vi "Main.vi"(11 "Module Admin":refnum<class "Delacor_lib_QMH_Module Admin.lvclass">) -> ()   [LabVIEW 2020, in "History.lvlib"]
doc: "This template is based off of the Queued Message Handler design pattern and the Queued Message Handler project template that ships with LabVIEW.\n\nThe main difference is that the queue is private to this module and communication between modules is performed via Broadcast and Request events.\n\nRequest events are wrapped in public API methods and are handled in the Event Handling Loop (EHL) of this VI. Any module can register for Broadcast events sent by this module. The EHL generates messages based on user interface actions.\n\nThe Message Handling Loop (MHL) processes messages generated by the EHL, or by other messages. The messages are string values, so new messages can be added easily to the Message Cases case structure in the MHL. Each message cluster can also provide an optional value for Message Data, which is a variant that can be converted to whatever message-specific data is required.\n_____\nBased on Delacor QMH Project Template 5.0.0.82."
uses:
  History.lvlib
  <vilib>/Delacor/Delacor QMH/Libraries/Module Admin_class/Delacor_lib_QMH_Module Admin.lvclass
  Module Data--cluster.ctl
  <vilib>/Delacor/Delacor QMH/Libraries/Message Queue_class/Delacor_lib_QMH_Message Queue.lvclass/Delacor_lib_QMH_Message Queue.ctl
  Stop Argument--cluster.ctl
  <vilib>/Delacor/Delacor QMH/Libraries/Module Admin_class/Delacor_lib_QMH_Module Admin.lvclass/Delacor_lib_QMH_Module Admin.ctl
  Agregar evento al historial Argument--cluster.ctl
  Mostrar en SubPanel Argument--cluster.ctl
  <vilib>/Delacor/Delacor QMH/Libraries/Message Queue_class/Delacor_lib_QMH_Enqueue Message (Single).vi
  <vilib>/Delacor/Delacor QMH/Libraries/Module Admin_class/Delacor_lib_QMH_Get External Launch.vi
  <vilib>/Utility/error.llb/Error Cluster From Error Code.vi
  <vilib>/ErrorRing/Error Ring.xnode
  <vilib>/Delacor/Delacor QMH/Libraries/Message Queue_class/Delacor_lib_QMH_Message Queue.lvclass
  <vilib>/Utility/miscctls.llb/LVPointTypeDef.ctl
panel:
  out "Multicolumn Listbox":i32(listbox)
  out "Lista de Eventos":string[](array[string])
  in  "CARGAR":bool
  in  "LIMPIAR":bool
  in  "Down Button":bool
  in  "Up Button":bool
  out "error out":errorcluster
  out "Status":string
  # "Histórico de Eventos"
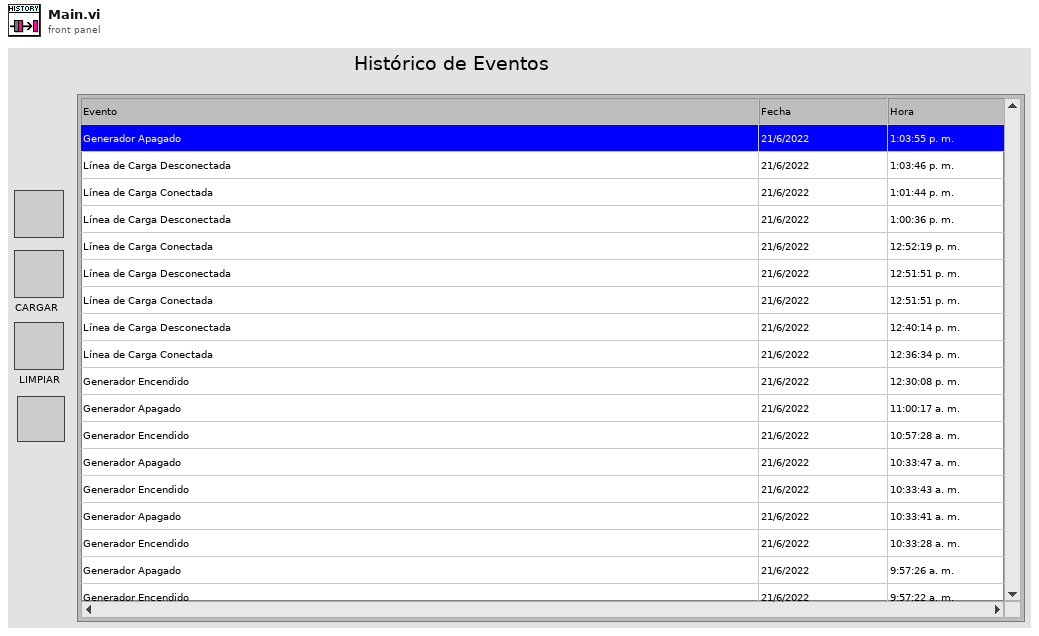
[diagram p1: front panel]
types:
  T1 = typedef "History.lvlib/Request Events--cluster.ctl" = cluster{"Stop Module":refnum<user-event>, "Show Panel":refnum<user-event>, "Hide Panel":refnum<user-event>, "Get Module Execution Status":refnum<user-event>, "Show Diagram":refnum<user-event>, "Agregar evento al historial":refnum<user-event>, "Mostrar en SubPanel":refnum<user-event>}
  T2 = typedef "History.lvlib/Module Data--cluster.ctl" = cluster{"Status":string}
  T3 = enum32{"invalid lock state", "Not Locked", "Locked (No Password)", "Password-protected"}
  T4 = typedef "History.lvlib/Stop Argument--cluster.ctl" = cluster{"Origin":string, "Exit via Stop Module Req?":bool, "Wait for Module to stop?":bool}
  T5 = typedef "History.lvlib/Agregar evento al historial Argument--cluster.ctl" = cluster{"Evento.valor":bool, "Evento.nombre":string}
  T6 = typedef "History.lvlib/Mostrar en SubPanel Argument--cluster.ctl" = cluster{"Subpanel Ref":refnum<vi>}
  T7 = enum32{"Invalid", "Standard", "Closed", "Hidden", "Minimized", "Maximized"}
  T8 = typedef "LVPointTypeDef.ctl" = cluster{"Horizontal":i16, "Vertical":i16}
  T9 = typedef "LVRowAndColumnUnsignedTypeDef.ctl" = cluster{"Row":u32, "Column":u32}
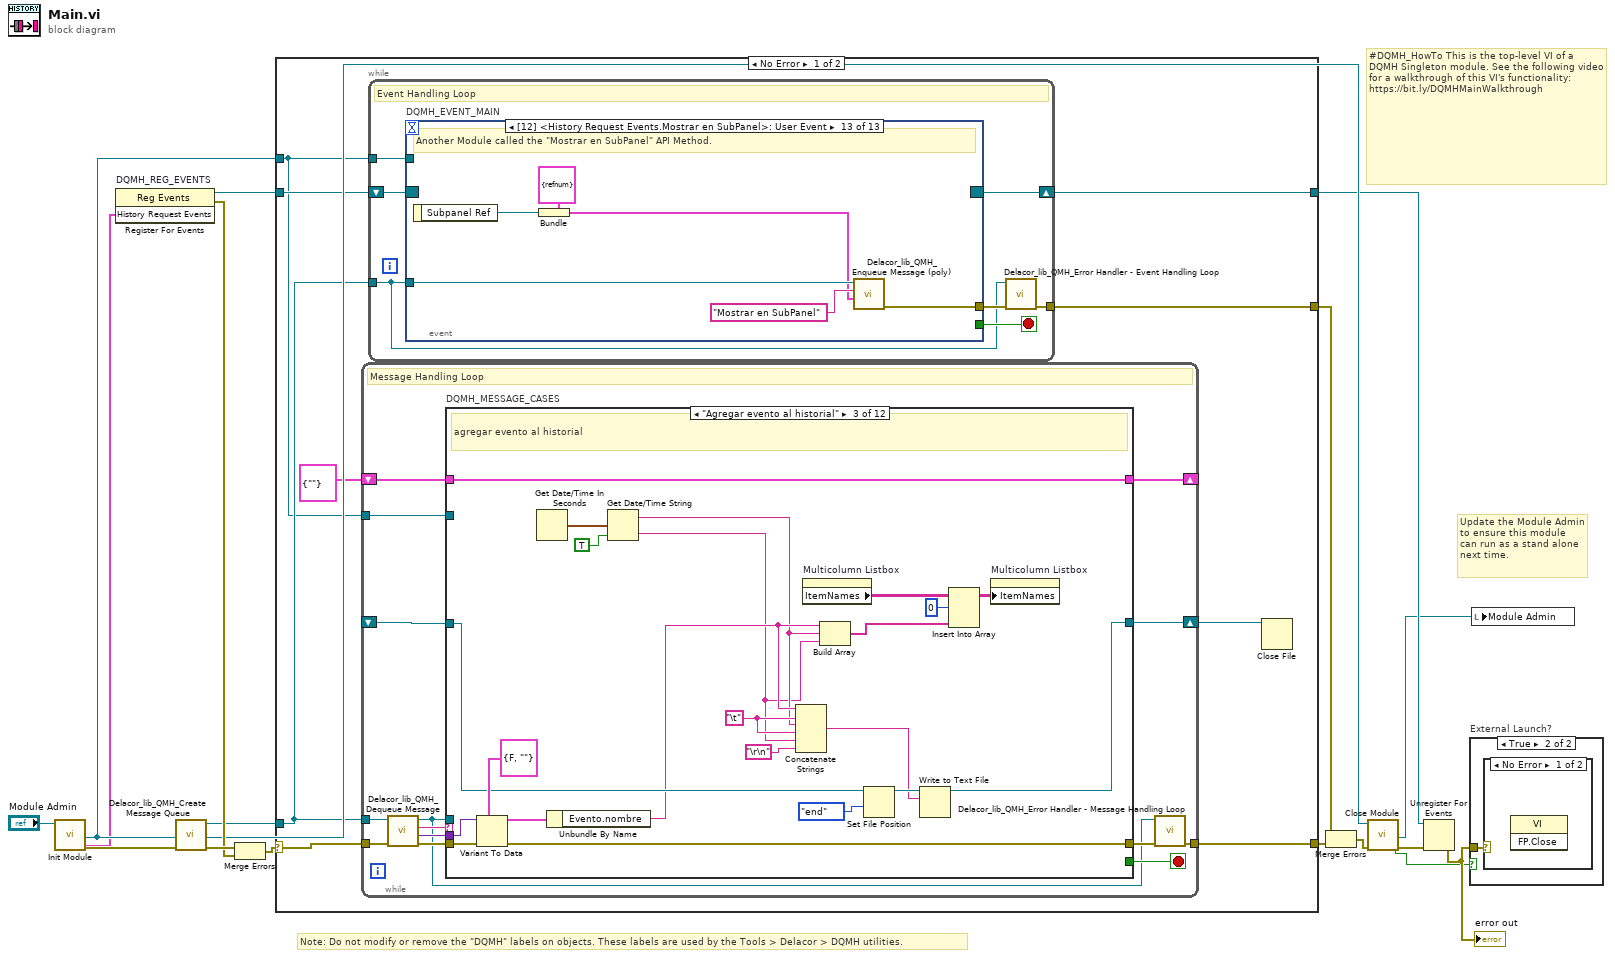
[diagram p0: block diagram]
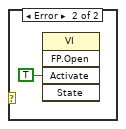
[diagram p3: hidden frame]
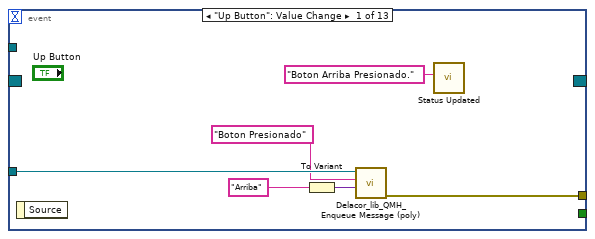
[diagram p4: hidden frame]
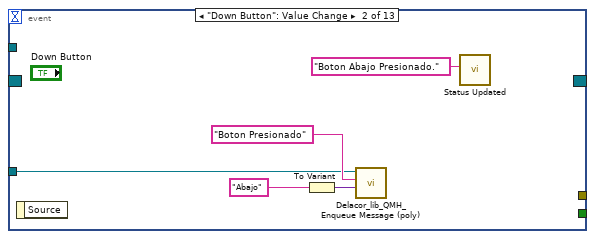
[diagram p5: hidden frame]
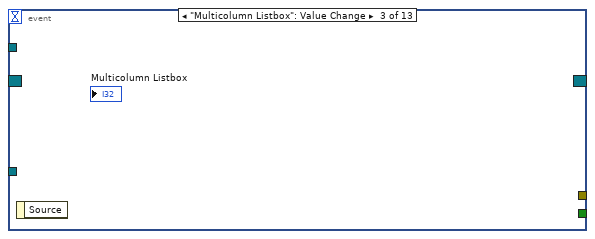
[diagram p6: hidden frame]
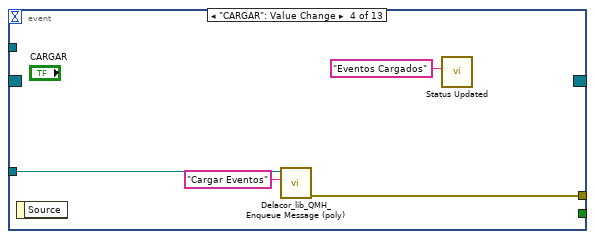
[diagram p7: hidden frame]
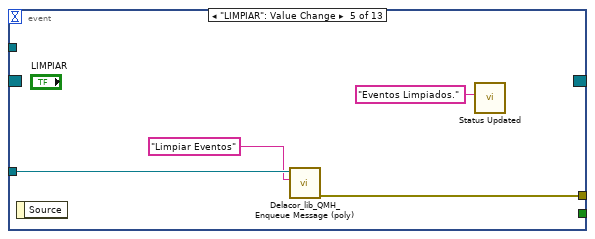
[diagram p8: hidden frame]
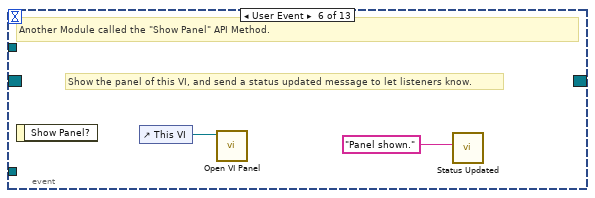
[diagram p9: hidden frame]
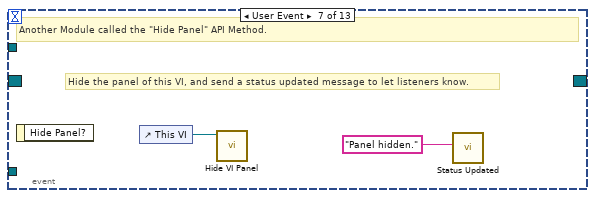
[diagram p10: hidden frame]
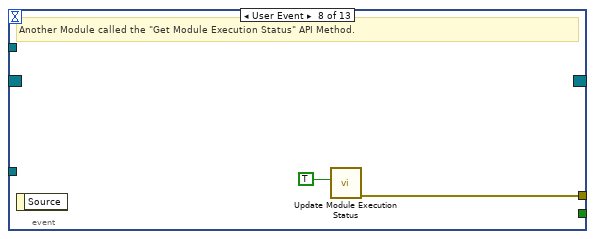
[diagram p11: hidden frame]
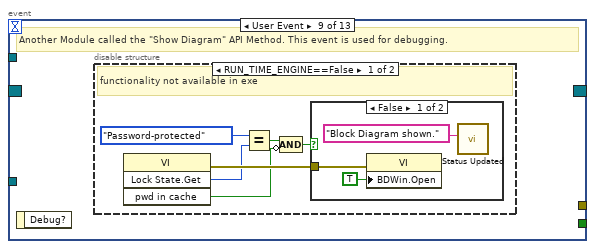
[diagram p12: hidden frame]
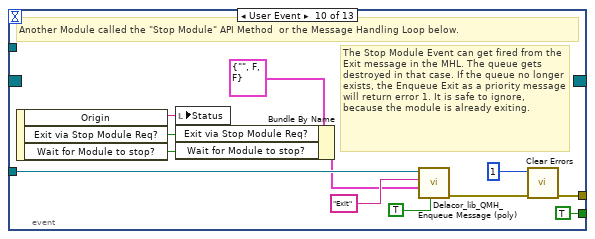
[diagram p15: hidden frame]
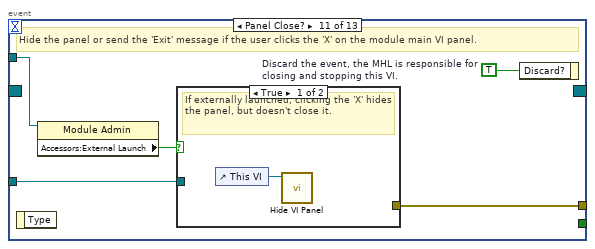
[diagram p16: hidden frame]
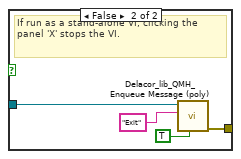
[diagram p17: hidden frame]
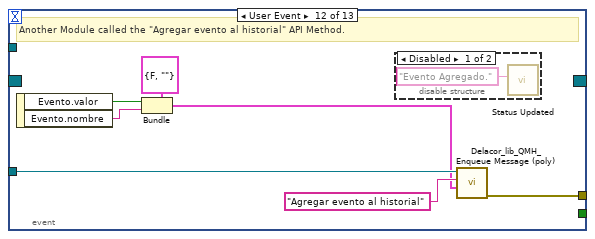
[diagram p18: hidden frame]
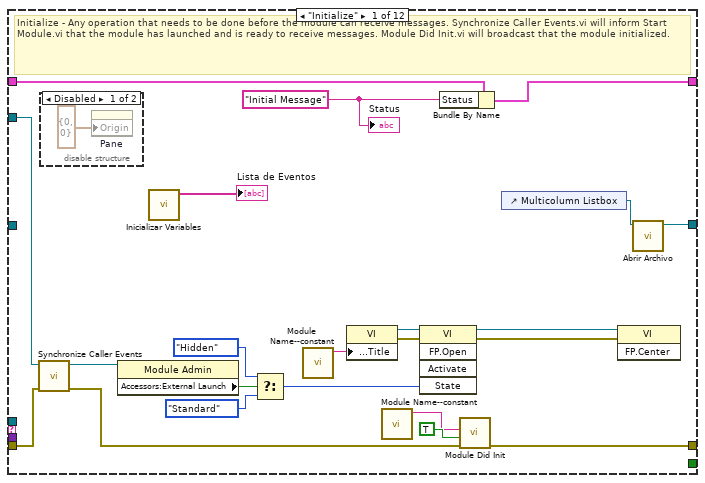
[diagram p20: hidden frame]
diagram:
  # "#DQMH_HowTo This is the top-level VI of a DQMH Singleton module. See the following video for a walkthrough of this VI's functionality: https://bit.ly/DQMHMainWalkthrough"
  # "Note: Do not modify or remove the \"DQMH\" labels on objects. These labels are used by the Tools > Delacor > DQMH utilities."
  # "Update the Module Admin to ensure this module can run as a stand alone next time."
  n1 = call "Init Module.vi"("Singleton Module Admin in"="Module Admin") -> ("error out"=w16:errorcluster, "History Request Events"=w5:T1, "Singleton Module Admin out"=w8:refnum<class "Delacor_lib_QMH_Module Admin.lvclass">)  [unwired: 8 in]
  n2 = register-events "DQMH_REG_EVENTS"(w5) -> (reference out=w6:refnum<event-registration>, error out=w9:errorcluster)  [unwired: 2 in]
  n3 = call <vilib>:"Delacor_lib_QMH_Create Message Queue.vi"("error in"=w16) -> ("error out"=w11:errorcluster, "Message Queue"=w4:refnum<class "Delacor_lib_QMH_Message Queue.lvclass">)  [unwired: 9 in]
  n4 = Merge Errors(w11, w9) -> (w10:errorcluster)
  n5 = case shown="No Error" w10 {
    selector: w10 -> [w24 w284]
    tunnel: [w26 w283] -> w17
    tunnel: [w23 w289] -> w7
    tunnel: w6 -> [w21 w289]
    tunnel: w4 -> [w20 w282]
    tunnel: [w25 _] -> w14
    tunnel: w8 -> [w19 w285]
    frame No Error {
      n6 = while {
        tunnel: w20 -> [w108]
        shift-right: [w112] -> _
        shift-left: T2 {"Status"=""} ("Data Cluster") -> [w113]
        tunnel: w24 -> [w116]
        tunnel: [w114] -> w26
        tunnel: w19 -> [w106]
        shift-right: [w105] -> w18
        shift-left: _ -> [w104]
        stop <- w111 stop-if-true
        # "Message Handling Loop"
        n7 = call-dynamic "Delacor_lib_QMH_Dequeue Message.vi"("error in"=w116, "Message Queue in"=w108) -> ("error out"=w115:errorcluster, "Message Data"=w109:variant, "Message"=w110:string, "Message Queue out"=w107:refnum<class "Delacor_lib_QMH_Message Queue.lvclass">)  [unwired: 6 in]
        n8 = case "DQMH_MESSAGE_CASES" shown="\"Agregar evento al historial\"" w110 {
          selector: w110 -> [_ _ _ _ _ _ _ _ _ _ _ w269]
          tunnel: w107 -> [_ _ _ _ _ _ _ _ _ w237 w260 _]
          tunnel: w115 -> [w137 w143 w165 w174 w178 w183 w190 w214 w232 w244 w266 w271]
          tunnel: [w135 w143 w163 w172 w177 w182 w189 w213 w232 w240 w263 w272] -> w117
          tunnel: w113 -> [w126 w142 w164 w173 w176 w181 w188 w212 w231 w239 w259 w270]
          tunnel: [w125 w142 w164 w173 w176 w181 w188 w212 w231 w239 w259 w270] -> w112
          tunnel: [_ _ _ _ _ _ _ _ _ _ w258 _] -> w111
          tunnel: w109 -> [_ _ w162 w171 _ _ _ w209 _ w238 w257 _]
          tunnel: w106 -> [w127 _ _ _ _ _ _ _ _ w236 w252 _]
          tunnel: [w118 w141 w147 _ w175 w180 w184 w211 w230 w233 w251 w267] -> w105
          tunnel: w104 -> [_ w141 w148 _ w175 w180 w186 w211 w230 w233 w251 w267]
          frame "Initialize" {
            w121 = "Initial Message" ("Initial Message")
            # "Initialize - Any operation that needs to be done before the module can receive messages. Synchronize Caller Events.vi will inform Start Module.vi that the module has launched and is ready to receive messages. Module Did Init.vi will broadcast that the module initialized."
            n9 = call "Synchronize Caller Events.vi"("error in (no error)"=w137, "Singleton Module Admin in"=w127) -> ("error out"=w136:errorcluster, "Singleton Module Admin out"=w122:refnum<class "Delacor_lib_QMH_Module Admin.lvclass">)  [unwired: 8 in]
            n10 = disable-structure shown="Disabled" {
              frame Disabled {
                n11 = property on="Pane" class="Pane"("Origin"=T8 {"Horizontal"=0, "Vertical"=0}) -> ()  [unwired: 2 in, 2 out]
              }
              frame Enabled {
              }
            }
            n12 = property class="Module Admin"(reference=w122) -> ("Accessors:External Launch"=w131:bool)  [unwired: 1 in, 2 out]
            n13 = call "Inicializar Variables.vi"() -> ("Lista de Eventos"=→"Lista de Eventos":string[])  [unwired: 11 in]
            n14 = Select(t=T7."Hidden" ("State"), s=w131, f=T7."Standard" ("State")) -> (s? t:f=w128:T7)
            n15 = call "Module Name--constant.vi"() -> ("Module Name"=w134:string)  [unwired: 11 in]
            n16 = property class="VI"("Front Panel.Title"=w134) -> (reference out=w133:refnum<vi>, error out=w139:errorcluster)  [unwired: 2 in]
            n17 = call "Module Name--constant.vi"() -> ("Module Name"=w123:string)  [unwired: 11 in]
            n18 = invoke class="VI" method="FP.Open"(reference=w133, error in=w139, "State"=w128) -> (reference out=w132:refnum<vi>, error out=w138:errorcluster)  [unwired: 2 in, 3 out]
            n19 = Bundle By Name(cluster=w126, "Status"=w121) -> (w125:T2)
            n20 = call "Module Did Init.vi"("error in (no error)"=w136, "Initialized?"=TRUE, "Origin"=w123) -> ("error out"=w135:errorcluster)  [unwired: 8 in]
            n21 = control-ref of="Multicolumn Listbox"() -> (w119:refnum<vi>)
            n22 = invoke class="VI" method="FP.Center"(reference=w132, error in=w138) -> ()  [unwired: 1 in, 3 out]
            n23 = call "Abrir Archivo.vi"("MulticolumnListbox in"=w119) -> ("Byte Stream File out"=w118:refnum<file>)  [unwired: 10 in]
            "Status" <- w121
          }
          frame "--- Module Specific ---" {
            # "Separator -- The following cases handle messages specific to this Module."
          }
          frame "Agregar evento al historial" {
            w151 = "\t"
            # "agregar evento al historial"
            n24 = Variant To Data(error in=w165, type=T5 {"Evento.valor"=FALSE, "Evento.nombre"=""} ("Agregar evento al historial Argument"), Variant=w162) -> (data=w160:T5, error out=w163:errorcluster)
            n25 = Get Date/Time In Seconds() -> (seconds since 1Jan1904=w159:timestamp)
            n26 = Unbundle By Name(w160) -> ("Evento.nombre"=w146:string)
            n27 = Get Date/Time String(seconds (now)=w159, want seconds? (F)=TRUE) -> (date string=w145:string, time string=w144:string)  [unwired: 1 in]
            n28 = Concatenate Strings(w146, w151, w145, w151, w144, "\r\n") -> (w153:string)
            n29 = property on="Multicolumn Listbox" class="MCListbox (strict)"() -> ("ItemNames"=w156:string[][])  [unwired: 2 in, 2 out]
            n30 = Build Array(w146, w145, w144) -> (w149:string[])
            n31 = Set File Position(refnum=w148, from (0:start)=enum16{"start", "end", "current"}."end") -> (refnum out=w154:refnum<file>)  [unwired: 2 in, 1 out]
            n32 = Write to Text File(file (use dialog)=w154, text=w153) -> (refnum out=w147:refnum<file>)  [unwired: 2 in, 2 out]
            n33 = Insert Into Array(array=w156, index (row)=0, new element=w149) -> (w155:string[][])  [unwired: 1 in]
            n34 = property on="Multicolumn Listbox" class="MCListbox (strict)"("ItemNames"=w155) -> ()  [unwired: 2 in, 2 out]
          }
          frame "Mostrar en SubPanel" {
            # "#CodeNeeded\n1. Configure this Message Case for handling the \"Mostrar en SubPanel\" message.\n2. Delete or edit this label when done."
            # "Mostrar el Módulo de Historial en el SubPanel del Main Module"
            n35 = Variant To Data(error in=w174, type=T6 {"Subpanel Ref"=refnum} ("Mostrar en SubPanel Argument"), Variant=w171) -> (data=w169:T6, error out=w172:errorcluster)
            n36 = Unbundle By Name(w169) -> ("Subpanel Ref"=w166:refnum<vi>)
            n37 = call "Module Name--constant.vi"() -> ("Module Name"=w167:string)  [unwired: 11 in]
            n38 = property class="VI"("Front Panel.Title"=w167) -> (reference out=w168:refnum<vi>)  [unwired: 2 in, 1 out]
            n39 = call "Insert SubPanel.vi"("VI Ref"=w168, "Subpanel Ref"=w166) -> ()  [unwired: 9 in, 1 out]
          }
          frame "---Copy This Frame---" {
            # "Duplicate this frame when creating new messages.  Change this comment in the duplicated frame to describe this message."
            n40 = Merge Errors(w178) -> (w177:errorcluster)
          }
          frame "Limpiar Eventos" {
            # "Duplicate this frame when creating new messages.  Change this comment in the duplicated frame to describe this message."
            n41 = property on="Multicolumn Listbox" class="MCListbox (strict)"("ItemNames"=string[][] [] ("Item Names")) -> ()  [unwired: 2 in, 2 out]
            n42 = Merge Errors(w183) -> (w182:errorcluster)
          }
          frame "Cargar Eventos" {
            # "Duplicate this frame when creating new messages.  Change this comment in the duplicated frame to describe this message."
            n43 = flat-sequence {
              tunnel: w186 -> [w193]
              tunnel: [w197] -> w187
              tunnel: [w191] -> w185
              tunnel: w187 -> [w203]
              tunnel: [w202] -> w184
              tunnel: w185 -> [w202]
              frame #0 {
                n44 = Set File Position(refnum=w193, from (0:start)=enum16{"start", "end", "current"}."start") -> (refnum out=w192:refnum<file>)  [unwired: 2 in, 1 out]
                n45 = Read from Text File(file (use dialog)=w192) -> (refnum out=w196:refnum<file>, text=w199:string)  [unwired: 2 in, 3 out]
                n46 = property on="Multicolumn Listbox" class="MCListbox (strict)"("ItemNames"=string[][] [] ("Array")) -> ()  [unwired: 2 in, 2 out]
                n47 = Spreadsheet String To Array(format string="%s", spreadsheet string=w199, array type (2D Dbl)=string[][] [] ("Array")) -> (array=w197:string[][])  [unwired: 1 in]
                n48 = Set File Position(refnum=w196, from (0:start)=enum16{"start", "end", "current"}."start") -> (refnum out=w191:refnum<file>)  [unwired: 2 in, 1 out]
              }
              frame #1 {
                n49 = for {
                  tunnel: w203 -> [w205] mode=indexing
                  n50 = property on="Multicolumn Listbox" class="MCListbox (strict)"() -> ("ItemNames"=w207:string[][])  [unwired: 2 in, 2 out]
                  n51 = Insert Into Array(array=w207, index (row)=0, new element=w205) -> (w206:string[][])  [unwired: 1 in]
                  n52 = property on="Multicolumn Listbox" class="MCListbox (strict)"("ItemNames"=w206) -> ()  [unwired: 2 in, 2 out]
                }
              }
            }
            n53 = Merge Errors(w190) -> (w189:errorcluster)
          }
          frame "Boton Presionado" {
            # "Duplicate this frame when creating new messages.  Change this comment in the duplicated frame to describe this message."
            n54 = Variant To Data(type="" ("Message"), Variant=w209) -> (data=w208:string)  [unwired: 1 in, 1 out]
            n55 = case shown="\"Abajo\", Default" w208 {
              frame "Abajo", Default {
                n56 = local read "Multicolumn Listbox"() -> (w218:i32)
                n57 = Greater?(x=w218, y=5) -> (0:w219:bool)
                n58 = case shown="True" w219 {
                  frame False {
                  }
                  frame True {
                    n59 = property on="Multicolumn Listbox" class="MCListbox (strict)"() -> ("TopLeft"=w222:T9)  [unwired: 2 in, 2 out]
                    n60 = Unbundle By Name(w222) -> ("Row"=w220:u32, "Column"=w224:u32)
                    n61 = Increment(x=w220) -> (x+1=w221:u32)
                    n62 = Bundle By Name(cluster=w222, "Row"=w221, "Column"=w224) -> (w223:T9)
                    n63 = property on="Multicolumn Listbox" class="MCListbox (strict)"("TopLeft"=w223) -> ()  [unwired: 2 in, 2 out]
                  }
                }
                n64 = Add(x=w218, y=1) -> (x+y=w217:i32)
                n65 = local write "Multicolumn Listbox"(w217) -> ()
              }
              frame "Arriba" {
                n66 = local read "Multicolumn Listbox"() -> (w226:i32)
                n67 = Equal To 0?(x=w226) -> (x = 0?=w229:bool)
                n68 = Subtract(x=w226, y=1) -> (x-y=w227:i32)
                n69 = Select(t=w226, s=w229, f=w227) -> (s? t:f=w228:i32)
                n70 = local write "Multicolumn Listbox"(w228) -> ()
              }
            }
            n71 = Merge Errors(w214) -> (w213:errorcluster)
          }
          frame "--- Exit and Error Handling---" {
            # "Separator - The following cases handle errors and exit messages."
          }
          frame "Error" {
            # "#CodeRecommended - If you ever change the name of this \"Error\" message, you'll need to update the name in the Check Loop Error.vi as well."
            # "#CodeRecommended - If the module is running in standalone mode (External Launch = FALSE), this code will pop up an error dialog and call the 'Exit' message if an error occurs. Add more fine-grained error handling here."
            # "Error - Check the error message data and respond accordingly. This message is sent by the \"Error Handler\" VIs at the end of each loop in this application."
            n72 = Variant To Data(error in=w244, type=errorcluster {"status"=FALSE, "code"=0, "source"=""} ("error constant"), Variant=w238) -> (data=w245:errorcluster, error out=w242:errorcluster)
            n73 = property class="Module Admin"(reference=w236) -> ("Accessors:External Launch"=w235:bool)  [unwired: 1 in, 2 out]
            n74 = call "Module Name--constant.vi"() -> ("Module Name"=w234:string)  [unwired: 11 in]
            n75 = call "Error Reported.vi"("Additional Information"=w234, "Error"=w245) -> ()  [unwired: 9 in, 1 out]
            n76 = case shown="False" w235 {
              tunnel: [w250 _] -> w241
              tunnel: w237 -> [w248 _]
              tunnel: w245 -> [w249 _]
              frame False {
                # "If the module is running standalone, then pop up an error dialog and call the \"Exit\" message."
                n77 = call <vilib>:"Simple Error Handler.vi"("error in (no error)"=w249) -> ()  [unwired: 4 in, 5 out]
                n78 = call-poly <vilib>:"Delacor_lib_QMH_Enqueue Message (poly).vi"("Priority Message? (F)"=TRUE, "Message"="Exit", "Message Queue in"=w248) -> ("error out"=w250:errorcluster)  [unwired: 7 in, 1 out]
              }
              frame True {
                # "If the module was launched externally, calling the Error Reported broadcast VI is the only action performed by the \"Error\" message. The module's caller can then process the error appropriately."
              }
            }
            n79 = Merge Errors(w242, w241) -> (w240:errorcluster)
            n80 = local write "error out"(w240) -> ()
          }
          frame "Exit" {
            w256 = 91  # 91: not all Exit messages will have an argument
            w258 = TRUE  # Stop the VI
            # "Release the message queue reference"
            # "#CodeNeeded - Add any required cleanup code here"
            # "Exit - Exit the application."
            n81 = Variant To Data(error in=w266, type=T4 {"Origin"="", "Exit via Stop Module Req?"=FALSE, "Wait for Module to stop?"=FALSE} ("Stop Argument"), Variant=w257) -> (data=w254:T4, error out=w262:errorcluster)
            n82 = call <vilib>:"Clear Errors.vi"("error in (no error)"=w262, "specific error code to clear (0: all)"=w256) -> ("error out"=w265:errorcluster)  [unwired: 4 in, 1 out]
            n83 = control-ref of="This VI"() -> (w253:refnum<vi>)
            n84 = call-dynamic "Delacor_lib_QMH_Release Message Queue.vi"("error in"=w265, "Message Queue"=w260) -> ("error out"=w264:errorcluster)  [unwired: 9 in]
            n85 = call "Handle Exit.vi"("Stop Argument"=w254, "Admin in"=w252, "VI reference"=w253) -> ("error out"=w261:errorcluster)  [unwired: 7 in, 1 out]
            n86 = Merge Errors(w264, w261) -> (w263:errorcluster)
          }
          frame Default {
            # "'Default' case only runs if there is a message that isn't defined in any of the other cases.  Output a programming error."
            n87 = call "Module Name--constant.vi"() -> ("Module Name"=w268:string)  [unwired: 11 in]
            n88 = xnode "Error Ring"("parameter 0"=w269, "parameter 1"=w268) -> ("error out"=w273:errorcluster)
            n89 = Merge Errors(w271, w273) -> (w272:errorcluster)
          }
        }
        n90 = call-dynamic "Delacor_lib_QMH_Error Handler - Message Handling Loop.vi"("error in"=w117, "Message Queue in"=w107) -> ("dup error in"=w114:errorcluster)  [unwired: 8 in, 1 out]
      }
      n91 = while {
        tunnel: w20 -> [w27]
        shift-right: [w30] -> w23
        shift-left: w21 -> [w31]
        tunnel: [w32] -> w25
        tunnel: w19 -> [w28]
        stop <- w29 stop-if-true
        # "Event Handling Loop"
        n92 = event "DQMH_EVENT_MAIN" shown="[12] <History Request Events.Mostrar en SubPanel>: User Event" {
          selector: w31 -> [_ _ _ _ _ _ _ _ _ _ _ _ _]
          dyn-events: [_ _ _ _ _ _ _ _ _ _ _ _ _] -> w30
          timeout: _ -> [_ _ _ _ _ _ _ _ _ _ _ _ _]
          tunnel: [_ _ _ _ _ _ _ _ _ TRUE ("Discard?") _ _ _] -> w29
          tunnel: w27 -> [w39 w41 _ w48 w51 _ _ _ _ w75 w82 w96 w103]
          tunnel: [w34 _ _ w45 w49 _ _ w58 _ w78 w84 w90 w98] -> w33
          tunnel: w28 -> [_ _ _ _ _ _ _ _ _ _ w81 _ _]
          event "Up Button": Value Change {
            n93 = event-data() -> ()  [unwired: 1 in, 1 out]
            n94 = To Variant(anything="Arriba" ("Message")) -> (Variant=w36:variant)
            n95 = call-poly <vilib>:"Delacor_lib_QMH_Enqueue Message (poly).vi"("Message Data"=w36, "Message"="Boton Presionado", "Message Queue in"=w39) -> ("error out"=w34:errorcluster)  [unwired: 7 in, 1 out]
            n96 = call "Status Updated.vi"("Status"="Boton Arriba Presionado.") -> ()  [unwired: 10 in, 1 out]
          }
          event "Down Button": Value Change {
            n97 = event-data() -> ()  [unwired: 1 in, 1 out]
            n98 = To Variant(anything="Abajo" ("Message")) -> (Variant=w44:variant)
            n99 = call-poly <vilib>:"Delacor_lib_QMH_Enqueue Message (poly).vi"("Message Data"=w44, "Message"="Boton Presionado", "Message Queue in"=w41) -> ()  [unwired: 7 in, 2 out]
            n100 = call "Status Updated.vi"("Status"="Boton Abajo Presionado.") -> ()  [unwired: 10 in, 1 out]
          }
          event "Multicolumn Listbox": Value Change {
            n101 = event-data() -> ()  [unwired: 1 in, 1 out]
          }
          event "CARGAR": Value Change {
            n102 = event-data() -> ()  [unwired: 1 in, 1 out]
            n103 = call-poly <vilib>:"Delacor_lib_QMH_Enqueue Message (poly).vi"("Message"="Cargar Eventos", "Message Queue in"=w48) -> ("error out"=w45:errorcluster)  [unwired: 8 in, 1 out]
            n104 = call "Status Updated.vi"("Status"="Eventos Cargados") -> ()  [unwired: 10 in, 1 out]
          }
          event "LIMPIAR": Value Change {
            n105 = event-data() -> ()  [unwired: 1 in, 1 out]
            n106 = call-poly <vilib>:"Delacor_lib_QMH_Enqueue Message (poly).vi"("Message"="Limpiar Eventos" ("Status"), "Message Queue in"=w51) -> ("error out"=w49:errorcluster)  [unwired: 8 in, 1 out]
            n107 = call "Status Updated.vi"("Status"="Eventos Limpiados.") -> ()  [unwired: 10 in, 1 out]
          }
          event User Event {
            # "Show the panel of this VI, and send a status updated message to let listeners know."
            # "Another Module called the \"Show Panel\" API Method."
            n108 = event-data() -> ()  [unwired: 1 in, 1 out]
            n109 = control-ref of="This VI"() -> (w54:refnum<vi>)
            n110 = call "Open VI Panel.vi"("VI"=w54) -> ()  [unwired: 10 in, 1 out]
            n111 = call "Status Updated.vi"("Status"="Panel shown." ("format string")) -> ()  [unwired: 10 in, 1 out]
          }
          event User Event {
            # "Hide the panel of this VI, and send a status updated message to let listeners know."
            # "Another Module called the \"Hide Panel\" API Method."
            n112 = event-data() -> ()  [unwired: 1 in, 1 out]
            n113 = control-ref of="This VI"() -> (w56:refnum<vi>)
            n114 = call "Hide VI Panel.vi"("VI"=w56) -> ()  [unwired: 10 in, 1 out]
            n115 = call "Status Updated.vi"("Status"="Panel hidden." ("format string")) -> ()  [unwired: 10 in, 1 out]
          }
          event User Event {
            # "Another Module called the \"Get Module Execution Status\" API Method."
            n116 = event-data() -> ()  [unwired: 1 in, 1 out]
            n117 = call "Update Module Execution Status.vi"("Running?"=TRUE) -> ("error out"=w58:errorcluster)  [unwired: 10 in]
          }
          event User Event {
            # "Another Module called the \"Show Diagram\" API Method. This event is used for debugging."
            n118 = event-data() -> ()  [unwired: 1 in, 1 out]
            n119 = disable-structure shown="RUN_TIME_ENGINE==False" {
              frame condition #0 (active) {
                # "functionality not available in exe"
                n120 = invoke class="VI" method="Lock State.Get"() -> (error out=w64:errorcluster, "Get Lock State"=w63:T3, "pwd in cache"=w60:bool)  [unwired: 4 in, 1 out]
                n121 = Equal?(x=T3."Password-protected", y=w63) -> (x = y?=w61:bool)
                n122 = Compound Arithmetic op=AND(w61, invert w60) -> (w59:bool)
                n123 = case shown="False" w59 {
                  tunnel: w64 -> [w67 _]
                  frame False {
                    n124 = property class="VI"(error in=w67, "BDWin.Open"=TRUE ("Block Diagram Window:Open")) -> ()  [unwired: 1 in, 2 out]
                    n125 = call "Status Updated.vi"("Status"="Block Diagram shown." ("format string")) -> ()  [unwired: 10 in, 1 out]
                  }
                  frame True {
                    # "Password-protected VI, and the password is not in the cache. Do not show the diagram."
                  }
                }
              }
              frame condition #1 {
              }
            }
          }
          event User Event {
            # "The Stop Module Event can get fired from the Exit message in the MHL. The queue gets destroyed in that case. If the queue no longer exists, the Enqueue Exit as a priority message will return error 1. It is safe to ignore, because the module is already exiting."
            # "Another Module called the \"Stop Module\" API Method  or the Message Handling Loop below."
            n126 = event-data() -> ("Origin"=w74:string, "Exit via Stop Module Req?"=w70:bool, "Wait for Module to stop?"=w69:bool)  [unwired: 1 in]
            n127 = local write "Status"(w74) -> ()
            n128 = Bundle By Name(cluster=T4 {"Origin"="", "Exit via Stop Module Req?"=FALSE, "Wait for Module to stop?"=FALSE} ("Stop Argument"), "Exit via Stop Module Req?"=w70, "Wait for Module to stop?"=w69) -> (w68:T4)
            n129 = call-poly <vilib>:"Delacor_lib_QMH_Enqueue Message (poly).vi"("Priority Message? (F)"=TRUE, "Message Data"=w68, "Message"="Exit", "Message Queue in"=w75) -> ("error out"=w79:errorcluster)  [unwired: 6 in, 1 out]
            n130 = call <vilib>:"Clear Errors.vi"("error in (no error)"=w79, "specific error code to clear (0: all)"=1) -> ("error out"=w78:errorcluster)  [unwired: 4 in, 1 out]
          }
          event Panel Close? {
            w83 = TRUE  # Discard the event, the MHL is responsible for closing and stopping this VI.
            # "Hide the panel or send the 'Exit' message if the user clicks the 'X' on the module main VI panel."
            n131 = event-data() -> ()  [unwired: 1 in, 1 out]
            n132 = property class="Module Admin"(reference=w81) -> ("Accessors:External Launch"=w80:bool)  [unwired: 1 in, 2 out]
            n133 = case shown="True" w80 {
              tunnel: w82 -> [_ w88]
              tunnel: [_ w89] -> w84
              frame True {
                # "If externally launched, clicking the 'X' hides the panel, but doesn't close it."
                n134 = control-ref of="This VI"() -> (w85:refnum<vi>)
                n135 = call "Hide VI Panel.vi"("VI"=w85) -> ()  [unwired: 10 in, 1 out]
              }
              frame False {
                # "If run as a stand-alone VI, clicking the panel 'X' stops the VI."
                n136 = call-poly <vilib>:"Delacor_lib_QMH_Enqueue Message (poly).vi"("Priority Message? (F)"=TRUE, "Message"="Exit", "Message Queue in"=w88) -> ("error out"=w89:errorcluster)  [unwired: 7 in, 1 out]
              }
            }
            n137 = event-data("Discard?"=w83) -> ()  [unwired: 1 in, 1 out]
          }
          event User Event {
            # "Another Module called the \"Agregar evento al historial\" API Method."
            n138 = event-data() -> ("Evento.valor"=w92:bool, "Evento.nombre"=w91:string)  [unwired: 1 in]
            n139 = Bundle(cluster=T5 {"Evento.valor"=FALSE, "Evento.nombre"=""} ("Agregar evento al historial Argument"), "Evento.valor"=w92, "Evento.nombre"=w91) -> (w93:T5)
            n140 = disable-structure shown="Disabled" {
              frame Disabled {
                n141 = call "Status Updated.vi"("Status"="Evento Agregado.") -> ()  [unwired: 10 in, 1 out]
              }
              frame Enabled {
              }
            }
            n142 = call-poly <vilib>:"Delacor_lib_QMH_Enqueue Message (poly).vi"("Message Data"=w93, "Message"="Agregar evento al historial", "Message Queue in"=w96) -> ("error out"=w90:errorcluster)  [unwired: 7 in, 1 out]
          }
          event User Event {
            # "Another Module called the \"Mostrar en SubPanel\" API Method."
            n143 = event-data() -> ("Subpanel Ref"=w99:refnum<vi>)  [unwired: 1 in]
            n144 = Bundle(cluster=T6 {"Subpanel Ref"=refnum} ("Mostrar en SubPanel Argument"), "Subpanel Ref"=w99) -> (w100:T6)
            n145 = call-poly <vilib>:"Delacor_lib_QMH_Enqueue Message (poly).vi"("Message Data"=w100, "Message"="Mostrar en SubPanel", "Message Queue in"=w103) -> ("error out"=w98:errorcluster)  [unwired: 7 in, 1 out]
          }
        }
        n146 = call-dynamic "Delacor_lib_QMH_Error Handler - Event Handling Loop.vi"("error in"=w33, "Message Queue in"=w27) -> ("dup error in"=w32:errorcluster)  [unwired: 8 in, 1 out]
      }
      n147 = Close File(refnum=w18) -> ()  [unwired: 1 in, 2 out]
    }
    frame Error {
      # "Synchronize Caller Events.vi will inform Start Module.vi that the module has launched and will let the code calling Start Module.vi register for broadcasts and would permit the caller receive the broadcast that an error occurred at launch time."
      n148 = call-dynamic "Delacor_lib_QMH_Release Message Queue.vi"("error in"=w284, "Message Queue"=w282) -> ("error out"=w283:errorcluster)  [unwired: 9 in]
      n149 = call "Synchronize Caller Events.vi"("Singleton Module Admin in"=w285) -> ("error out"=w290:errorcluster)  [unwired: 9 in, 1 out]
      n150 = call "Module Name--constant.vi"() -> ("Module Name"=w288:string)  [unwired: 11 in]
      n151 = Format Into String(format string="An error occurred during initialization. %s is no longer running.", w288) -> (resulting string=w286:string)  [unwired: 2 in, 1 out]
      n152 = Merge Errors(w283, w290) -> (w291:errorcluster)
      n153 = call "Error Reported.vi"("Additional Information"=w286, "Error"=w291) -> ()  [unwired: 9 in, 1 out]
    }
  }
  n154 = Merge Errors(w14, w17) -> (w13:errorcluster)
  n155 = call "Close Module.vi"("error in (no error)"=w13, "Module Admin in"=w8) -> ("error out"=w15:errorcluster, "External Launch"=w1:bool, "Module Admin out"=w2:refnum<class "Delacor_lib_QMH_Module Admin.lvclass">)  [unwired: 7 in]
  n156 = Unregister For Events(event registration refnum=w7, error in=w15) -> (error out=w12:errorcluster)
  "error out" <- w12
  n157 = case "External Launch?" shown="True" w1 {
    tunnel: w12 -> [_ w292]
    frame False {
    }
    frame True {
      n158 = case shown="No Error" w292 {
        frame No Error {
          n159 = invoke class="VI" method="FP.Close"() -> ()  [unwired: 3 in, 3 out]
        }
        frame Error {
          n160 = invoke class="VI" method="FP.Open"("Activate"=TRUE ("Activate?")) -> ()  [unwired: 4 in, 5 out]
        }
      }
    }
  }
  n161 = local write "Module Admin"(w2) -> ()
